vi "Compute Link Transform.vi"(8 "error in (no error)":errorcluster, 10 "q":dbl, 11 "Link in":refnum<class "NI_Robotics_Link.lvclass">) -> (0 "error out":errorcluster, 2 "Link Transform":T1, 3 "Link out":refnum<class "NI_Robotics_Link.lvclass">)   [LabVIEW 2017, in "NI_Robotics_Link.lvclass"]
uses:
  <vilib>/robotics/Kinematics/Link/NI_Robotics_Link.lvclass
  <vilib>/Analysis/Matrix/Datatypes/RealMatrix.ctl
  <vilib>/robotics/Kinematics/Link/NI_Robotics_Link.lvclass/NI_Robotics_Link.ctl
  <vilib>/Analysis/Matrix/NI_Matrix.lvlib
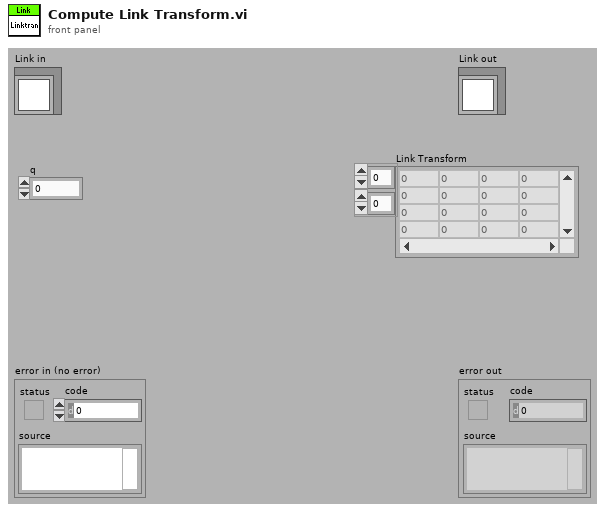
[diagram p1: front panel]
types:
  T1 = typedef "NI_Matrix.lvlib/RealMatrix.ctl" = dbl[][]
  T2 = typedef "NI_Robotics_Link.lvclass/Joint Type.ctl" = enum16{"Revolute", "Prismatic"}
  T3 = typedef "NI_Kinematics.lvlib/DH Convention.ctl" = enum16{"Standard", "Modified"}
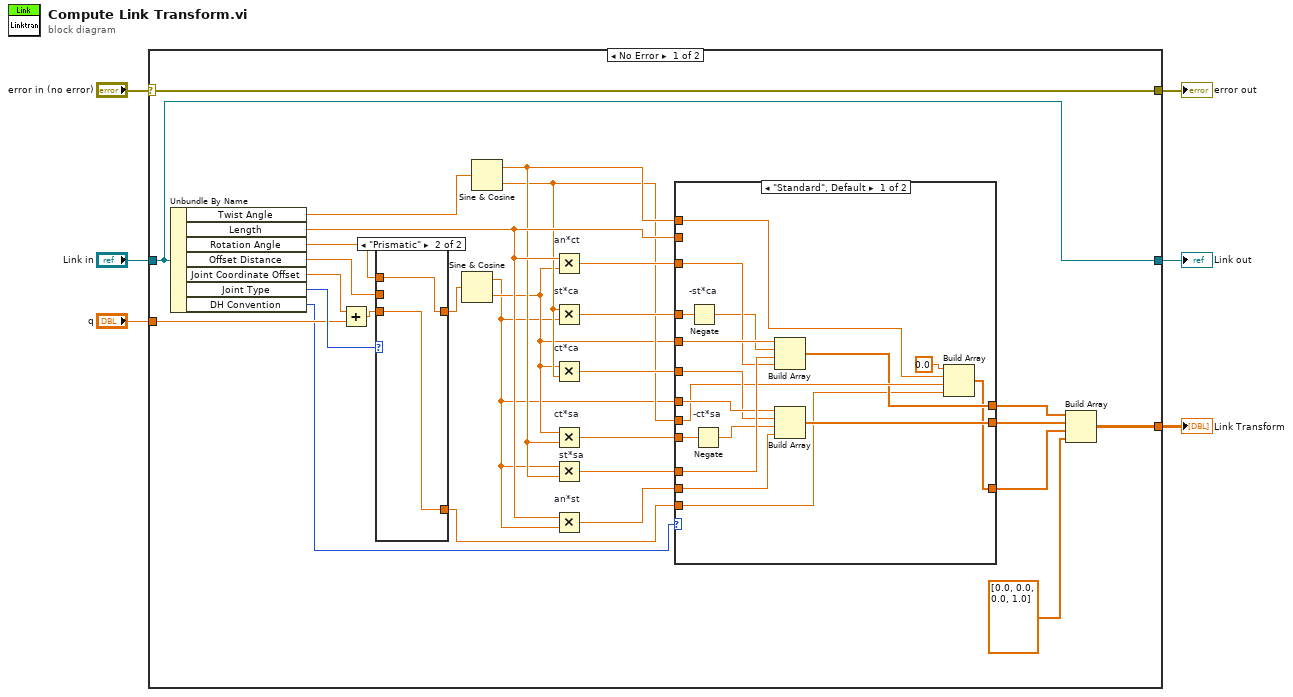
[diagram p0: block diagram]
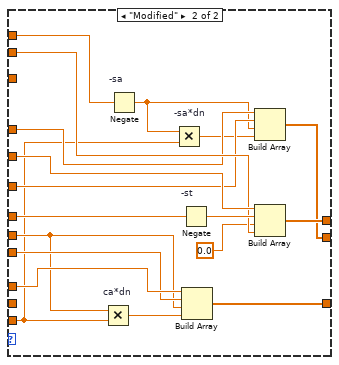
[diagram p2: hidden frame]
diagram:
  n1 = case shown="No Error" "error in (no error)" {
    selector: "error in (no error)" -> [w34 w75]
    tunnel: [w34 w75] -> w5
    tunnel: [w33 w74] -> w3
    tunnel: "Link in" -> [w33 w74]
    tunnel: "q" -> [w24 _]
    tunnel: [w13 _] -> w1
    frame No Error {
      n2 = Unbundle By Name(w33) -> ("Twist Angle"=w12:dbl, "Length"=w17:dbl, "Rotation Angle"=w21:dbl, "Offset Distance"=w20:dbl, "Joint Coordinate Offset"=w23:dbl, "Joint Type"=w25:T2, "DH Convention"=w18:T3)
      n3 = Add(x=w23, y=w24) -> (x+y=w22:dbl)
      n4 = case shown="\"Prismatic\"" w25 {
        tunnel: w21 -> [_ w73]
        tunnel: w22 -> [w71 w72]
        tunnel: [w71 w73] -> w7
        tunnel: w20 -> [w70 _]
        tunnel: [w70 w72] -> w19
        frame "Revolute", Default {
        }
        frame "Prismatic" {
        }
      }
      n5 = Sine & Cosine(0:w7) -> (1:w8:dbl, 2:w9:dbl)
      n6 = Sine & Cosine(0:w12) -> (1:w11:dbl, 2:w10:dbl)
      n7 = Multiply "an*ct"(x=w17, y=w9) -> (x*y=w31:dbl)
      n8 = Multiply "st*ca"(x=w10, y=w8) -> (x*y=w16:dbl)
      n9 = Multiply "ct*ca"(x=w9, y=w10) -> (x*y=w30:dbl)
      n10 = Multiply "ct*sa"(x=w9, y=w11) -> (x*y=w15:dbl)
      n11 = Multiply "st*sa"(x=w8, y=w11) -> (x*y=w32:dbl)
      n12 = Multiply "an*st"(x=w17, y=w8) -> (x*y=w29:dbl)
      n13 = case shown="\"Standard\", Default" w18 {
        tunnel: w9 -> [w51 w69]
        tunnel: w32 -> [w50 w57]
        tunnel: w31 -> [w49 _]
        tunnel: w8 -> [w48 w68]
        tunnel: w30 -> [w47 w62]
        tunnel: w29 -> [w46 _]
        tunnel: w11 -> [w44 w61]
        tunnel: w10 -> [w43 w55]
        tunnel: [w42 w64] -> w28
        tunnel: [w41 w58] -> w27
        tunnel: [w40 w52] -> w26
        tunnel: w19 -> [w39 w54]
        tunnel: w17 -> [_ w66]
        tunnel: w16 -> [w36 w63]
        tunnel: w15 -> [w37 w56]
        frame "Standard", Default {
          n14 = Negate "-st*ca"(x=w36) -> (-x=w35:dbl)
          n15 = Negate "-ct*sa"(x=w37) -> (-x=w38:dbl)
          n16 = Build Array(w51, w35, w50, w49) -> (w42:dbl[])
          n17 = Build Array(w48, w47, w38, w46) -> (w41:dbl[])
          n18 = Build Array(0.0 ("element"), w44, w43, w39) -> (w40:dbl[])
        }
        frame "Modified" {
          n19 = Multiply "ca*dn"(x=w55, y=w54) -> (x*y=w53:dbl)
          n20 = Negate "-sa"(x=w61) -> (-x=w60:dbl)
          n21 = Multiply "-sa*dn"(x=w60, y=w54) -> (x*y=w59:dbl)
          n22 = Negate "-st"(x=w68) -> (-x=w67:dbl)
          n23 = Build Array(w57, w56, w55, w53) -> (w52:dbl[])
          n24 = Build Array(w63, w62, w60, w59) -> (w58:dbl[])
          n25 = Build Array(w69, w67, 0.0 ("element"), w66) -> (w64:dbl[])
        }
      }
      n26 = Build Array(w28, w27, w26, dbl[] [0.0, 0.0, 0.0, 1.0]) -> (w13:dbl[][])
    }
    frame Error {
    }
  }
  "error out" <- w5
  "Link out" <- w3
  "Link Transform" <- w1
